vi "Ex1-Calling the python-hello.vi"() -> ()   [LabVIEW 2021]
uses:
  <vilib>/httpClient/LabVIEWHTTPClient.lvlib
panel:
  in  "Cluster Error":cluster{"error":string}={"error"="Rate limit exceeded: 5 per 1 minute"}
  in  "Cluster":cluster{"status":string, "text":string}={"status"="success", "text"="Hello"}
  out "body":string="{\"error\":\"Rate limit exceeded: 5 per 1 minute\"}"
  out "headers":string="HTTP/1.1 429 Too Many Requests\r\ndate: Mon, 02 Mar 2026 11:39:28 GMT\r\nserver: uvicorn\r\ncontent-length: 47\r\ncontent-type: application/json\r\n\r\n"
  in  "url":string="http://localhost:8080/calling"
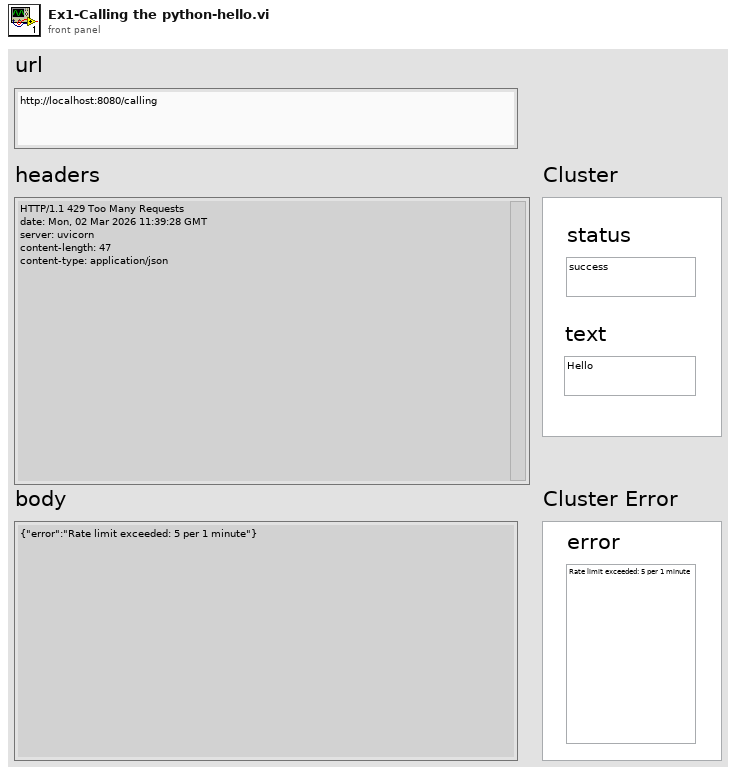
[diagram p1: front panel]
types:
  T1 = typedef "LabVIEWHTTPClient.lvlib/ClientHandle.ctl" = refnum<k1>
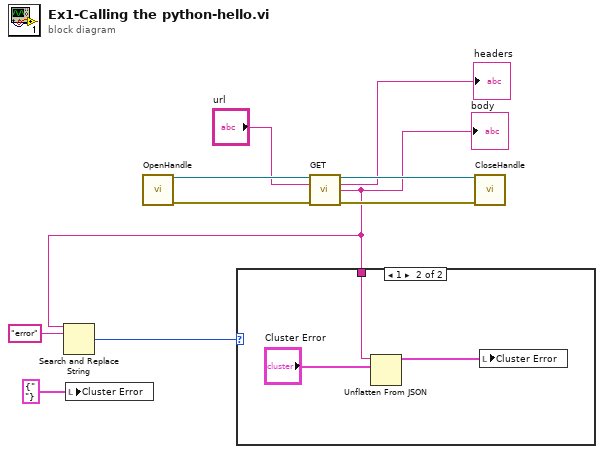
[diagram p0: block diagram]
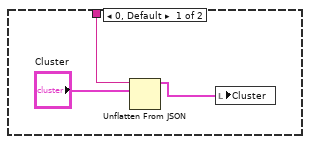
[diagram p2: hidden frame]
diagram:
  n1 = local write "Cluster Error"(cluster{"error":string} {"error"=" "} ("Cluster Error")) -> ()
  n2 = call <vilib>:"OpenHandle.vi"() -> ("client handle out"=w10:T1, "error out"=w9:errorcluster)  [unwired: 14 in]
  n3 = call <vilib>:"GET.vi"("client handle"=w10, "url"="url", "error in (no error)"=w9) -> ("client handle out"=w8:T1, "headers"=→"headers":string, "body"=w3:string, "error out"=w7:errorcluster)  [unwired: 9 in]
  "body" <- w3
  n4 = Search and Replace String(input string=w3, search string="error") -> (number of replacements=w4:i32)  [unwired: 6 in, 3 out]
  n5 = case shown="1" w4 {
    tunnel: w3 -> [w12 w15]
    frame 0, Default {
      n6 = Unflatten From JSON(JSON string=w12, type and defaults="Cluster") -> (value=w11:cluster{"status":string, "text":string})  [unwired: 5 in, 1 out]
      n7 = local write "Cluster"(w11) -> ()
    }
    frame 1 {
      n8 = Unflatten From JSON(JSON string=w15, type and defaults="Cluster Error") -> (value=w14:cluster{"error":string})  [unwired: 5 in, 1 out]
      n9 = local write "Cluster Error"(w14) -> ()
    }
  }
  n10 = call <vilib>:"CloseHandle.vi"("client handle"=w8, "error in (no error)"=w7) -> ()  [unwired: 13 in, 1 out]
